vi "Acknowledge Faults.vi"(0 "object in":refnum<class "PowerModuleInterface.lvclass">, 11 "Error In":errorcluster) -> (4 "object out":refnum<class "PowerModuleInterface.lvclass">, 15 "Error Out":errorcluster)   [LabVIEW 2023, in "PowerModuleInterface.lvlib" / "PowerModuleInterface.lvclass"]
uses:
  PowerModuleInterface.lvclass
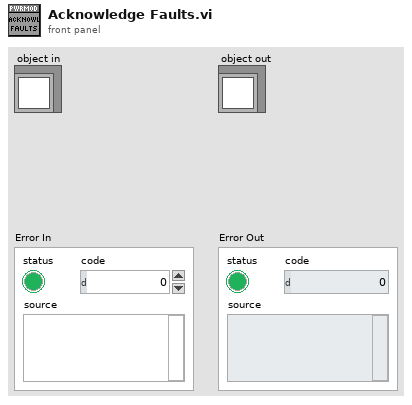
[diagram p1: front panel]
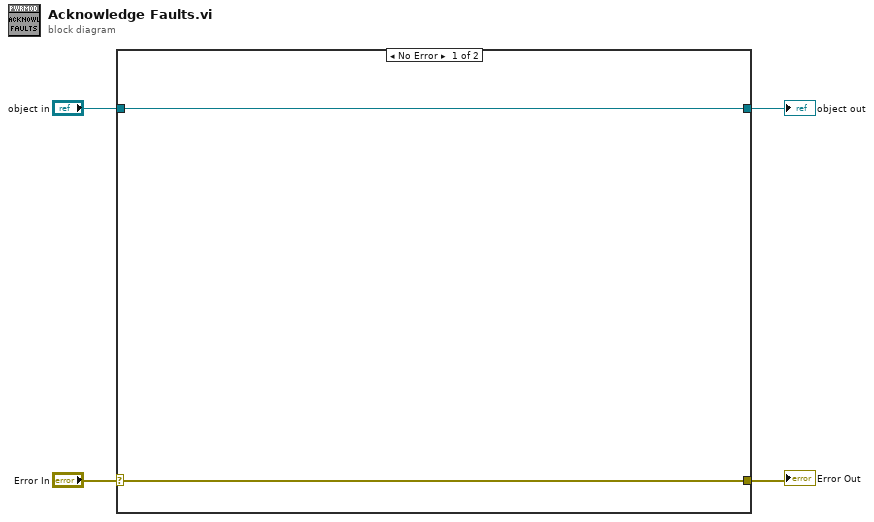
[diagram p0: block diagram]
diagram:
  n1 = case shown="No Error" "Error In" {
    selector: "Error In" -> [w6 w8]
    tunnel: [w6 w8] -> w3
    tunnel: [w5 w7] -> w1
    tunnel: "object in" -> [w5 w7]
    frame No Error {
    }
    frame Error {
    }
  }
  "Error Out" <- w3
  "object out" <- w1
